vi "DropDetection.vi"(8 "error in":errorcluster, 11 "Path":path) -> (0 "error out":errorcluster, 1 "Image Out":T1(plugin-control), 2 "Particle Measurements (Pixels)":dbl[][](array[numeric]) format="%.2f", 3 "Number of Particles":i32)   [LabVIEW 2013]
uses:
  <vilib>/vision/NI_Vision_Development_Module.lvlib
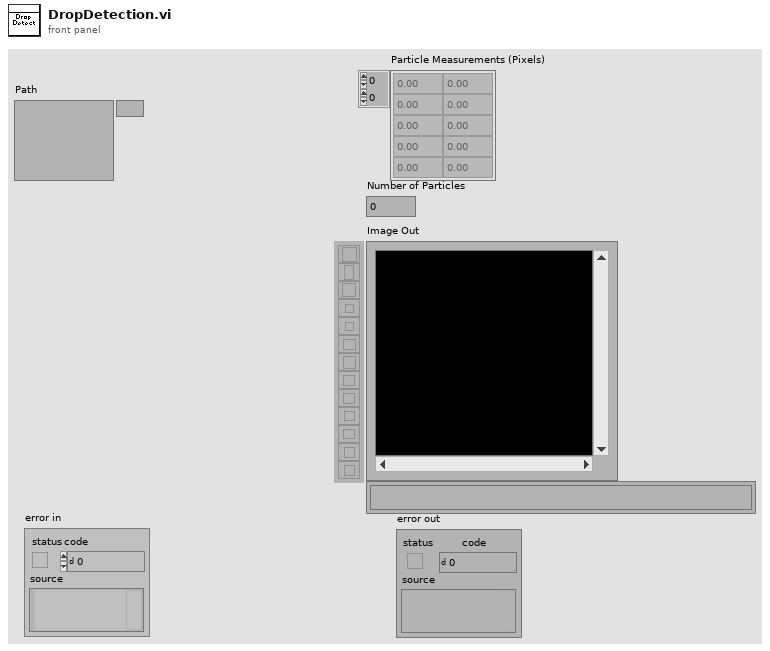
[diagram p1: front panel]
types:
  T1 = typedef "IMAQ Image.ctl" = refnum<image>
  T2 = enum32{"AutoM", "Close", "Dilate", "Erode", "Gradient", "Gradient out", "Gradient in", "Hit miss", "Open", "PClose", "POpen", "Thick", "Thin"}
  T3 = cluster{"Measurement Parameter":i32, "Range Lower Value":dbl, "Range Upper Value":dbl, "Range":bool, "Measurement Type":bool}[]
  T4 = cluster{"Registration Method":u32, "Normalization Method":u32, "Edge Thickness to Ignore":i32, "Bright Threshold":sgl, "Dark Threshold":sgl, "Grayscale/ Binary?":bool}
  T5 = typedef "Image Type" = u32
  T6 = cluster{"Transformed point":cluster{"Left":sgl, "Top":sgl}, "Transformed Angle":sgl, "Numeric out":dbl}
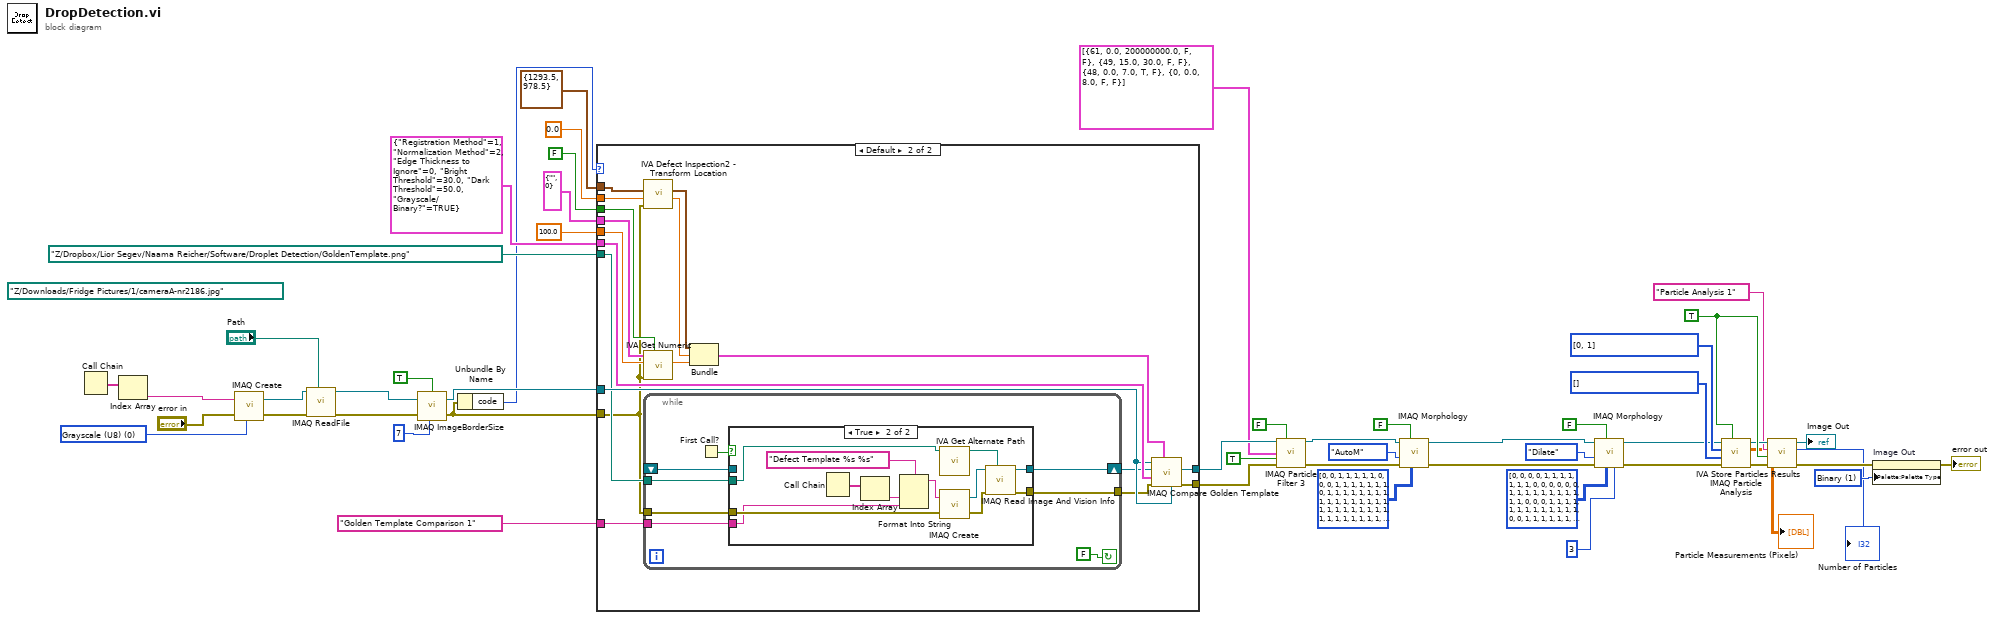
[diagram p0: block diagram]
diagram:
  (unwired) path "Z:/Downloads/Fridge Pictures/1/cameraA-nr2186.jpg" ("Path")
  w6 = u32 1 items=["Grayscale", "Binary", "Gradient", "Rainbow", "Temperature", "User Defined"] ("Palette")
  w14 = i32[] [] items=["Center of Mass X", "Center of Mass Y", "First Pixel X", "First Pixel Y", "Bounding Rect Left", "Bounding Rect Top", "Bounding Rect Right", "Bounding Rect Bottom", "Max Feret Diameter Start X", "Max Feret Diameter Start Y", "Max Feret Diameter End X", "Max Feret Diameter End Y", "Max Horiz. Segment Length Left", "Max Horiz. Segment Length Right", "Max Horiz. Segment Length Row", "-", "Bounding Rect Width", "Bounding Rect Height", "Bounding Rect Diagonal", "Perimeter", "Convex Hull Perimeter", "Holes' Perimeter", "Max Feret Diameter", "Equivalent Ellipse Major Axis", "Equivalent Ellipse Minor Axis", "Equivalent Ellipse Minor Axis (Feret)", "Equivalent Rect Long Side", "Equivalent Rect Short Side", "Equivalent Rect Diagonal", "Equivalent Rect Short Side (Feret)", "Average Horiz. Segment Length", "Average Vert. Segment Length", "Hydraulic Radius", "Waddel Disk Diameter", "-", "Area", "Holes' Area", "Particle & Holes' Area", "Convex Hull Area", "Image Area", "-", "Number of Holes", "Number of Horiz. Segments", "Number of Vert. Segments", "-", "Orientation", "Max Feret Diameter Orientation", "-", "% Area/Image Area", "% Area/(Particle & Holes' Area)", "Ratio of Equivalent Ellipse Axes", "Ratio of Equivalent Rect Sides", "-", "Elongation Factor", "Compactness Factor", "Heywood Circularity Factor", "Type Factor", "-", "Sum X", "Sum Y", "Sum XX", "Sum XY", "Sum YY", "Sum XXX", "Sum XXY", "Sum XYY", "Sum YYY", "-", "Moment of Inertia XX", "Moment of Inertia XY", "Moment of Inertia YY", "Moment of Inertia XXX", "Moment of Inertia XXY", "Moment of Inertia XYY", "Moment of Inertia YYY", "Norm. Moment of Inertia XX", "Norm. Moment of Inertia XY", "Norm. Moment of Inertia YY", "Norm. Moment of Inertia XXX", "Norm. Moment of Inertia XXY", "Norm. Moment of Inertia XYY", "Norm. Moment of Inertia YYY", "Hu Moment 1", "Hu Moment 2", "Hu Moment 3", "Hu Moment 4", "Hu Moment 5", "Hu Moment 6", "Hu Moment 7"] ("Real-World Measurements")
  w15 = i32[] [0, 1] items=["Center of Mass X", "Center of Mass Y", "First Pixel X", "First Pixel Y", "Bounding Rect Left", "Bounding Rect Top", "Bounding Rect Right", "Bounding Rect Bottom", "Max Feret Diameter Start X", "Max Feret Diameter Start Y", "Max Feret Diameter End X", "Max Feret Diameter End Y", "Max Horiz. Segment Length Left", "Max Horiz. Segment Length Right", "Max Horiz. Segment Length Row", "-", "Bounding Rect Width", "Bounding Rect Height", "Bounding Rect Diagonal", "Perimeter", "Convex Hull Perimeter", "Holes' Perimeter", "Max Feret Diameter", "Equivalent Ellipse Major Axis", "Equivalent Ellipse Minor Axis", "Equivalent Ellipse Minor Axis (Feret)", "Equivalent Rect Long Side", "Equivalent Rect Short Side", "Equivalent Rect Diagonal", "Equivalent Rect Short Side (Feret)", "Average Horiz. Segment Length", "Average Vert. Segment Length", "Hydraulic Radius", "Waddel Disk Diameter", "-", "Area", "Holes' Area", "Particle & Holes' Area", "Convex Hull Area", "Image Area", "-", "Number of Holes", "Number of Horiz. Segments", "Number of Vert. Segments", "-", "Orientation", "Max Feret Diameter Orientation", "-", "% Area/Image Area", "% Area/(Particle & Holes' Area)", "Ratio of Equivalent Ellipse Axes", "Ratio of Equivalent Rect Sides", "-", "Elongation Factor", "Compactness Factor", "Heywood Circularity Factor", "Type Factor", "-", "Sum X", "Sum Y", "Sum XX", "Sum XY", "Sum YY", "Sum XXX", "Sum XXY", "Sum XYY", "Sum YYY", "-", "Moment of Inertia XX", "Moment of Inertia XY", "Moment of Inertia YY", "Moment of Inertia XXX", "Moment of Inertia XXY", "Moment of Inertia XYY", "Moment of Inertia YYY", "Norm. Moment of Inertia XX", "Norm. Moment of Inertia XY", "Norm. Moment of Inertia YY", "Norm. Moment of Inertia XXX", "Norm. Moment of Inertia XXY", "Norm. Moment of Inertia XYY", "Norm. Moment of Inertia YYY", "Hu Moment 1", "Hu Moment 2", "Hu Moment 3", "Hu Moment 4", "Hu Moment 5", "Hu Moment 6", "Hu Moment 7"] ("Pixel Measurements")
  w11 = TRUE ("Connectivity 4/8 (8)")
  w47 = T5 0 items=["Grayscale (U8)", "Grayscale (I16)", "Grayscale (SGL)", "Complex (CSG)", "RGB (U32)", "HSL (U32)", "RGB (U64)", "Grayscale (U16)"] ("Image Type")
  n1 = Call Chain() -> (call chain=w49:string[])
  n2 = Index Array(array=w49) -> (element=w48:string)  [unwired: 1 in]
  n3 = call "IMAQ Create"("Image Name"=w48, "Image Type"=w47, "error in (no error)"="error in") -> ("New Image"=w52:T1, "error out"=w51:errorcluster)  [unwired: 1 in, 1 out]
  n4 = call "IMAQ ReadFile"("File Path"="Path", "error in (no error)"=w51, "Image"=w52) -> ("error out"=w45:errorcluster, "Image Out"=w46:T1)  [unwired: 2 in, 5 out]
  n5 = call "IMAQ ImageBorderSize"("Get/Set Status? (Set)"=TRUE, "Image"=w46, "Image border size in"=7 ("Border Size"), "error in (no error)"=w45) -> ("Image Out"=w35:T1, "error out"=w34:errorcluster)  [unwired: 1 out]
  n6 = Unbundle By Name(w34) -> ("code"=w33:i32)
  n7 = case shown="Default" w33 {
    tunnel: path "Z:/Dropbox/Lior Segev/Naama Reicher/Software/Droplet Detection/GoldenTemplate.png" ("Template File Path") -> [_ w59]
    tunnel: T4 {"Registration Method"=1, "Normalization Method"=2, "Edge Thickness to Ignore"=0, "Bright Threshold"=30.0, "Dark Threshold"=50.0, "Grayscale/ Binary?"=TRUE} ("Inspection Options") -> [_ w71]
    tunnel: [_ w55] -> w28
    tunnel: [w53 w70] -> w29
    tunnel: 100.0 ("Scale") -> [_ w69]
    tunnel: cluster{"GUID":string, "Index":i32} {"GUID"="", "Index"=0} ("Scale ID") -> [_ w68]
    tunnel: FALSE ("Scale Source") -> [_ w67]
    tunnel: cluster{"x":sgl, "y":sgl} {"x"=1293.5, "y"=978.5} ("Position") -> [_ w64]
    tunnel: sgl 0.0 ("Angle") -> [_ w63]
    tunnel: w34 -> [_ w56]
    tunnel: w35 -> [w53 w60]
    tunnel: "Golden Template Comparison 1" ("Step Name") -> [_ w54]
    frame -1074396199, -1074396198 {
      # "Discard Coordinate System Error"
    }
    frame Default {
      n8 = call <vilib>:"IVA Defect Inspection2 - Transform Location.vi"("error in (no error)"=w56, "Angle"=w63, "Point"=w64) -> ("Transformed Angle"=w61:sgl, "Transformed point"=w62:cluster{"Left":sgl, "Top":sgl})  [unwired: 1 in, 6 out]
      n9 = call <vilib>:"IVA Get Numeric.vi"("Source"=w67, "error in"=w56, "Numeric in"=w69, "Result ID"=w68) -> ("Numeric out"=w66:dbl)  [unwired: 7 out]
      n10 = while {
        shift-right: [w78] -> w58
        shift-left: _ -> [w77]
        tunnel: [w75] -> w57
        tunnel: w56 -> [w74]
        tunnel: w59 -> [w73]
        tunnel: w54 -> [w72]
        stop <- FALSE continue-if-true
        n11 = First Call?() -> (First Call?: T/F=w79:bool)
        n12 = case shown="True" w79 {
          tunnel: [w81 w91] -> w78
          tunnel: w77 -> [w81 _]
          tunnel: [w80 w88] -> w75
          tunnel: w74 -> [w80 w87]
          tunnel: w73 -> [_ w84]
          tunnel: w72 -> [_ w82]
          frame False {
          }
          frame True {
            n13 = Call Chain() -> (call chain=w86:string[])
            n14 = Index Array(array=w86) -> (element=w85:string)  [unwired: 1 in]
            n15 = Format Into String(format string="Defect Template %s %s" ("Image Name"), w85, w82) -> (resulting string=w93:string)  [unwired: 2 in, 1 out]
            n16 = call <vilib>:"IVA Get Alternate Path.vi"("Path In"=w84) -> ("Path Out"=w83:path)  [unwired: 10 out]
            n17 = call "IMAQ Create"("Image Name"=w93, "error in (no error)"=w87) -> ("New Image"=w90:T1, "error out"=w89:errorcluster)  [unwired: 2 in, 1 out]
            n18 = call "IMAQ Read Image And Vision Info"("File Path"=w83, "error in (no error)"=w89, "Image"=w90) -> ("error out"=w88:errorcluster, "Image Out"=w91:T1)  [unwired: 1 in, 6 out]
          }
        }
      }
      n19 = Bundle("Transformed point"=w62, "Transformed Angle"=w61, "Numeric out"=w66) -> (w65:T6)  [unwired: 1 out]
      n20 = call "IMAQ Compare Golden Template"("Dark Defect Image Dst"=w60, "Alignment"=w65, "error in (no error)"=w57, "Inspection Options"=w71, "Template Image"=w58, "Image"=w60) -> ("error out"=w55:errorcluster, "Dark Defect Image Dst Out"=w70:T1)  [unwired: 1 in, 3 out]
    }
  }
  n21 = call "IMAQ Particle Filter 3"("Image Src"=w29, "Connectivity 4/8 (8)"=FALSE, "Selection Values"=T3 [{"Measurement Parameter"=61, "Range Lower Value"=0.0, "Range Upper Value"=200000000.0, "Range"=FALSE, "Measurement Type"=FALSE}, {"Measurement Parameter"=49, "Range Lower Value"=15.0, "Range Upper Value"=30.0, "Range"=FALSE, "Measurement Type"=FALSE}, {"Measurement Parameter"=48, "Range Lower Value"=0.0, "Range Upper Value"=7.0, "Range"=TRUE, "Measurement Type"=FALSE}, {"Measurement Parameter"=0, "Range Lower Value"=0.0, "Range Upper Value"=8.0, "Range"=FALSE, "Measurement Type"=FALSE}], "Keep/Remove Particles (F)"=TRUE ("Keep/Remove Particles"), "error in (no error)"=w28) -> ("Image Dst Out"=w23:T1, "error out"=w22:errorcluster)  [unwired: 4 in, 5 out]
  n22 = call "IMAQ Morphology"("Structuring Element"=i32[][] [[0, 0, 1, 1, 1, 1, 1, 0, 0], [0, 1, 1, 1, 1, 1, 1, 1, 0], [1, 1, 1, 1, 1, 1, 1, 1, 1], [1, 1, 1, 1, 1, 1, 1, 1, 1], [1, 1, 1, 1, 1, 1, 1, 1, 1], [1, 1, 1, 1, 1, 1, 1, 1, 1], [1, 1, 1, 1, 1, 1, 1, 1, 1], [0, 1, 1, 1, 1, 1, 1, 1, 0], [0, 0, 1, 1, 1, 1, 1, 0, 0]], "Square/Hexa (Square)"=FALSE, "error in (no error)"=w22, "Operation"=T2."AutoM", "Image Src"=w23) -> ("error out"=w16:errorcluster, "Image Dst Out"=w17:T1)  [unwired: 2 in, 3 out]
  n23 = call "IMAQ Morphology"("Number of iterations (1)"=3, "Structuring Element"=i32[][] [[0, 0, 0, 0, 1, 1, 1, 1, 1, 1, 1, 0, 0, 0, 0], [0, 0, 1, 1, 1, 1, 1, 1, 1, 1, 1, 1, 1, 0, 0], [0, 1, 1, 1, 1, 1, 1, 1, 1, 1, 1, 1, 1, 1, 0], [0, 1, 1, 1, 1, 1, 1, 1, 1, 1, 1, 1, 1, 1, 0], [1, 1, 1, 1, 1, 1, 1, 1, 1, 1, 1, 1, 1, 1, 1], [1, 1, 1, 1, 1, 1, 1, 1, 1, 1, 1, 1, 1, 1, 1], [1, 1, 1, 1, 1, 1, 1, 1, 1, 1, 1, 1, 1, 1, 1], [1, 1, 1, 1, 1, 1, 1, 1, 1, 1, 1, 1, 1, 1, 1], [1, 1, 1, 1, 1, 1, 1, 1, 1, 1, 1, 1, 1, 1, 1], [1, 1, 1, 1, 1, 1, 1, 1, 1, 1, 1, 1, 1, 1, 1], [1, 1, 1, 1, 1, 1, 1, 1, 1, 1, 1, 1, 1, 1, 1], [0, 1, 1, 1, 1, 1, 1, 1, 1, 1, 1, 1, 1, 1, 0], [0, 1, 1, 1, 1, 1, 1, 1, 1, 1, 1, 1, 1, 1, 0], [0, 0, 1, 1, 1, 1, 1, 1, 1, 1, 1, 1, 1, 0, 0], [0, 0, 0, 0, 1, 1, 1, 1, 1, 1, 1, 0, 0, 0, 0]], "Square/Hexa (Square)"=FALSE, "error in (no error)"=w16, "Operation"=T2."Dilate", "Image Src"=w17) -> ("error out"=w13:errorcluster, "Image Dst Out"=w12:T1)  [unwired: 1 in, 3 out]
  n24 = call "IMAQ Particle Analysis"("Connectivity 4/8 (8)"=w11, "error in (no error)"=w13, "Real-World Measurements"=w14, "Pixel Measurements"=w15, "Image"=w12) -> ("error out"=w8:errorcluster, "Particle Measurements (Pixels)"=→"Particle Measurements (Pixels)":dbl[][], "Image Out (duplicate)"=w10:T1)  [unwired: 4 out]
  n25 = call <vilib>:"IVA Store Particles Results.vi"("error in (no error)"=w8, "Connectivity 4/8 (8)"=w11, "Step Name"="Particle Analysis 1", "Image in"=w10) -> ("error out"=w5:errorcluster, "Number of Particles"=→"Number of Particles":i32, "Image dup"=→"Image Out":T1)  [unwired: 5 out]
  n26 = property on="Image Out" class="ImageControl"(error in=w5, "Palette:Palette Type"=w6) -> (error out=→"error out":errorcluster)  [unwired: 1 in, 1 out]
